vi "Select_int.vi"(8 "False":cluster{i16, i16, i16, i16, i16, i16, i16, i16}, 10 "Input":T1, 11 "True":cluster{i16, i16, i16, i16, i16, i16, i16, i16}) -> (2 "output":cluster{i16, i16, i16, i16, i16, i16, i16, i16})   [LabVIEW 2017]
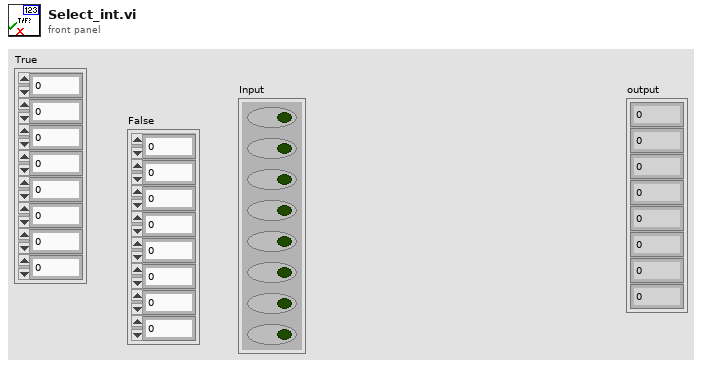
[diagram p1: front panel]
types:
  T1 = cluster{bool, bool, bool, bool, bool, bool, bool, bool}
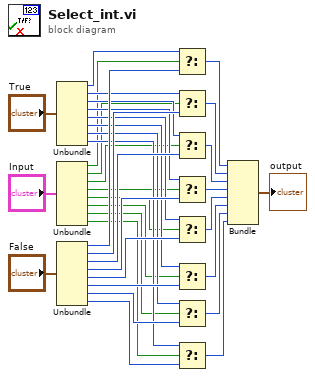
[diagram p0: block diagram]
diagram:
  n1 = Unbundle("True") -> (w13:i16, w14:i16, w15:i16, w16:i16, w17:i16, w18:i16, w19:i16, w20:i16)
  n2 = Unbundle("Input") -> (w11:bool, w10:bool, w9:bool, w8:bool, w7:bool, w6:bool, w5:bool, w4:bool)
  n3 = Unbundle("False") -> (w21:i16, w22:i16, w23:i16, w24:i16, w25:i16, w26:i16, w27:i16, w28:i16)
  n4 = Select(t=w13, s=w11, f=w21) -> (s? t:f=w36:i16)
  n5 = Select(t=w14, s=w10, f=w22) -> (s? t:f=w35:i16)
  n6 = Select(t=w15, s=w9, f=w23) -> (s? t:f=w34:i16)
  n7 = Select(t=w16, s=w8, f=w24) -> (s? t:f=w33:i16)
  n8 = Select(t=w17, s=w7, f=w25) -> (s? t:f=w32:i16)
  n9 = Select(t=w18, s=w6, f=w26) -> (s? t:f=w31:i16)
  n10 = Select(t=w19, s=w5, f=w27) -> (s? t:f=w30:i16)
  n11 = Select(t=w20, s=w4, f=w28) -> (s? t:f=w29:i16)
  n12 = Bundle(w36, w35, w34, w33, w32, w31, w30, w29) -> (→"output":cluster{i16, i16, i16, i16, i16, i16, i16, i16})  [unwired: 1 in]
